vi "SENS_CORR_EXT_REC_R_TIME_OBSOLETE.vi"(0 "VISA IN":refnum<visa-resource-name>, 1 "Receiver":i32, 2 "Length(sec)":i32, 5 "error in":errorcluster, 7 "Channel":i32) -> (14 "VISA Out":refnum<visa-resource-name>, 19 "error out":errorcluster)   [LabVIEW 2018, in "PNA-X.lvlib"]
doc: "SENSe<cnum>:CORRection:EXTension:RECeiver<Rnum>[:TIME] <num> OBSOLETE \n(Read-Write) This command has NO replacement and no longer works. \nSets the extension value at the specified receiver. Must also set SENS:CORR:EXT ON. \nNote: Before using this command you must select a measurement using CALC:PAR:SEL. You can \nselect one measurement for each channel. \nParameters \n<cnum> Any existing channel number. If unspecified, value is set to 1 \n<Rnum> Number of the receiver that will receive the extension. If unspecified, value is \nset to 1 \nChoose from: \n1 for Receiver A \n2 for Receiver B \n<num> The electrical length in seconds; may include suffix. Choose a number \nbetween: \n-10 and 10 \nExamples SENS:CORR:EXT:REC 2MS \nsense2:correction:extension:receiver2:time .00025 \nQuery Syntax SENSe<cnum>:CORRection:EXTension:RECeiver<Rnum> [:TIME]? \n1707\n\nReturn Type Numeric \nDefault 0"
uses:
  PNA-X.lvlib
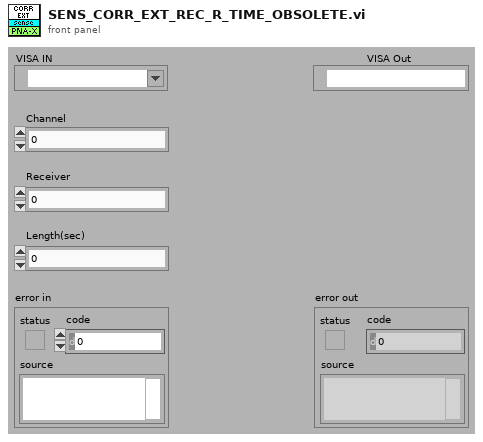
[diagram p1: front panel]
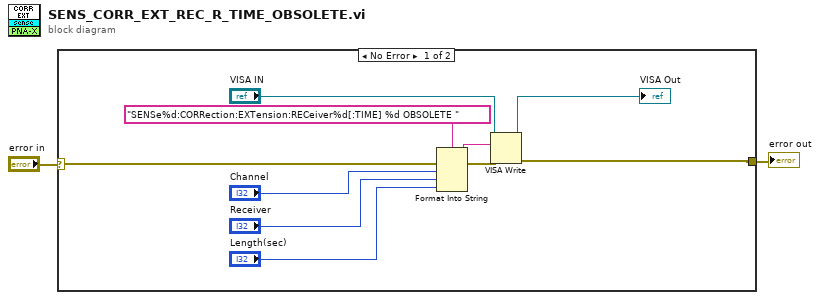
[diagram p0: block diagram]
diagram:
  n1 = case shown="No Error" "error in" {
    selector: "error in" -> [w12 w13]
    tunnel: [w7 w13] -> w1
    frame No Error {
      n2 = Format Into String(format string="SENSe%d:CORRection:EXTension:RECeiver%d[:TIME] %d OBSOLETE " ("Cmdline"), error in=w12, "Channel", "Receiver", "Length(sec)") -> (resulting string=w10:string, error out=w11:errorcluster)  [unwired: 1 in]
      n3 = VISA Write(VISA resource name="VISA IN", write buffer=w10, error in (no error)=w11) -> (VISA resource name out=→"VISA Out":refnum<visa-resource-name>, error out=w7:errorcluster)  [unwired: 1 out]
    }
    frame Error {
    }
  }
  "error out" <- w1
